vi "MotorMultiAbsolu.vi"(3 "Motors":string[](array[string]), 4 "Positions":i32[](array[numeric]), 9 "error in (no error)":errorcluster) -> (0 "Motors out":string[](array[string]), 1 "Ok?":refnum<k4>[](array[refnum]), 6 "error out":errorcluster)   [LabVIEW 2009]
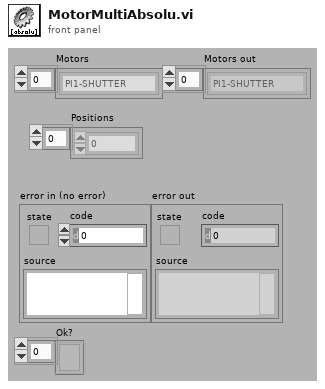
[diagram p1: front panel]
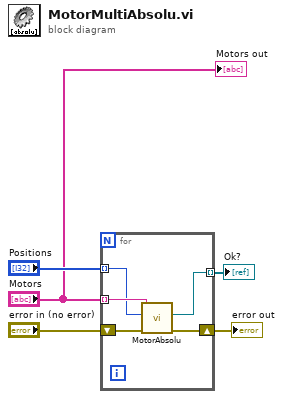
[diagram p0: block diagram]
diagram:
  n1 = for {
    tunnel: "Positions" -> [w7] mode=indexing
    tunnel: "Motors" -> [w8] mode=indexing
    shift-right: [w9] -> w3
    shift-left: "error in (no error)" -> [w10]
    tunnel: [w6] -> w1 mode=indexing
    n2 = call "MotorAbsolu.vi"("Motor"=w8, "Position"=w7, "error in (no error)"=w10) -> ("Ok?"=w6:refnum<k4>, "error out"=w9:errorcluster)  [unwired: 4 in, 1 out]
  }
  "error out" <- w3
  "Ok?" <- w1
  "Motors out" <- "Motors"
